vi "ConfigureSimulatedData.vi"() -> ()   [LabVIEW 2017, in "IrAcquisition.lvlib"]
uses:
  <vilib>/addons/InsightCM/Devices/Shared/Ir/IrAcquisition/IrAcquisition.lvlib
  <vilib>/addons/InsightCM/Devices/Shared/Ir/IrAcquisition/controls/simScaleConfig.ctl
  <vilib>/addons/InsightCM/Devices/Shared/Ir/IrAcquisition/subVIs/SimConfigGlobal.vi
panel:
  in  "Camera 2 Data":string(combo)
  in  "Camera 2 SN":string="67890DEF"
  in  "Camera 2 Config":T1={"Max"={"Enable"=FALSE, "New Max Temp"=100.0, "KeepMin"=FALSE}, "Noise"={"Randomize"=TRUE, "Max delta"=0.5}, "Hotspot"={"hotspot"=FALSE, "Rectangle"={"left"=100, "top"=200, "right"=150, "bottom"=250}, "Temperature"=100.0}}
  in  "Camera 1 Data":string(combo)
  in  "Camera 1 SN":string="12345ABC"
  in  "Camera 1 Config":T1={"Max"={"Enable"=FALSE, "New Max Temp"=100.0, "KeepMin"=FALSE}, "Noise"={"Randomize"=TRUE, "Max delta"=0.5}, "Hotspot"={"hotspot"=FALSE, "Rectangle"={"left"=100, "top"=200, "right"=150, "bottom"=250}, "Temperature"=100.0}}
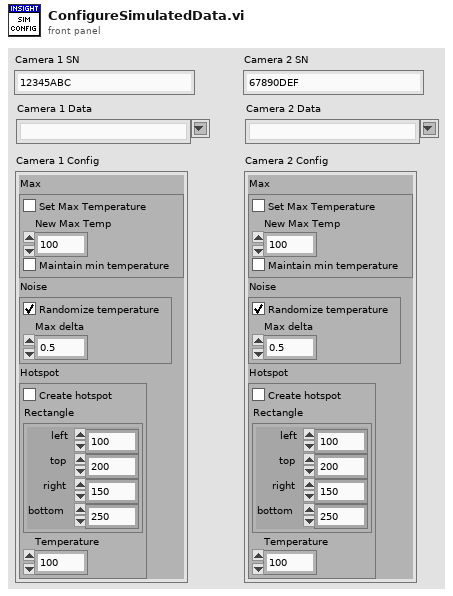
[diagram p1: front panel]
types:
  T1 = typedef "IrAcquisition.lvlib/simScaleConfig.ctl" = cluster{"Max":cluster{"Enable":bool, "New Max Temp":sgl, "KeepMin":bool}, "Noise":cluster{"Randomize":bool, "Max delta":sgl}, "Hotspot":cluster{"hotspot":bool, "Rectangle":cluster{"left":i16, "top":i16, "right":i16, "bottom":i16}, "Temperature":sgl}}
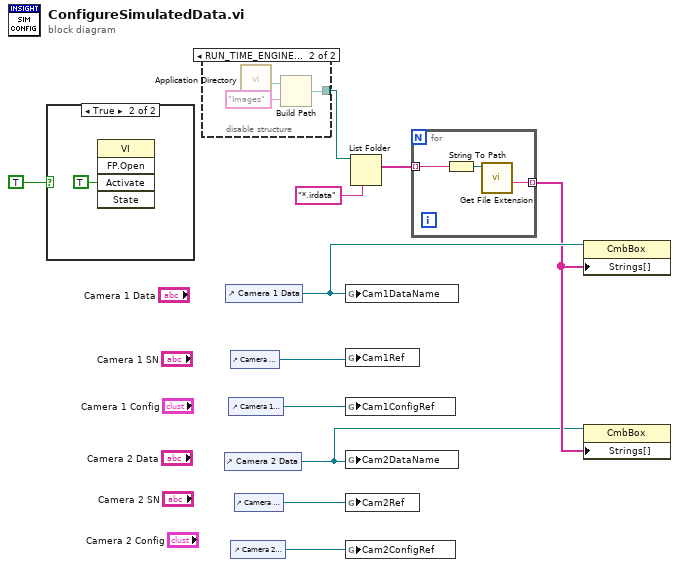
[diagram p0: block diagram]
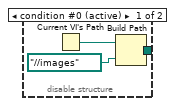
[diagram p2: hidden frame]
diagram:
  n1 = case shown="True" TRUE {
    frame False {
    }
    frame True {
      n2 = invoke class="VI" method="FP.Open"("Activate"=TRUE ("Activate?")) -> ()  [unwired: 4 in, 5 out]
    }
  }
  n3 = disable-structure shown="RUN_TIME_ENGINE==True" {
    disable-tunnel: [w13 w16] -> w8
    frame condition #0 (active) {
      n4 = Current VI's Path() -> (path=w15:path)
      n5 = Build Path(base path=w15, name or relative path=path "../../images" ("path")) -> (appended path=w13:path)
    }
    frame condition #1 {
      n6 = call <vilib>:"Application Directory.vi"() -> ("Application Directory"=w18:path)
      n7 = Build Path(base path=w18, name or relative path="Images") -> (appended path=w16:path)
    }
  }
  n8 = control-ref of="Camera 2 Data"() -> (w3:refnum<vi>)
  n9 = control-ref of="Camera 1 Data"() -> (w5:refnum<vi>)
  n10 = control-ref of="Camera 1 Config"() -> (w9:refnum<vi>)
  n11 = control-ref of="Camera 1 SN"() -> (w10:refnum<vi>)
  n12 = control-ref of="Camera 2 Config"() -> (w1:refnum<vi>)
  n13 = control-ref of="Camera 2 SN"() -> (w2:refnum<vi>)
  n14 = global write "SimConfigGlobal.vi" "Cam1DataName"(w5) -> ()
  n15 = global write "SimConfigGlobal.vi" "Cam1Ref"(w10) -> ()
  n16 = global write "SimConfigGlobal.vi" "Cam1ConfigRef"(w9) -> ()
  n17 = global write "SimConfigGlobal.vi" "Cam2DataName"(w3) -> ()
  n18 = global write "SimConfigGlobal.vi" "Cam2Ref"(w2) -> ()
  n19 = global write "SimConfigGlobal.vi" "Cam2ConfigRef"(w1) -> ()
  n20 = List Folder(path=w8, pattern="*.irdata") -> (filenames=w6:string[])  [unwired: 2 in, 3 out]
  n21 = for {
    tunnel: w6 -> [w21] mode=indexing
    tunnel: [w19] -> w4 mode=indexing
    n22 = String To Path(string=w21) -> (path=w20:path)
    n23 = call <vilib>:"Get File Extension.vi"("file"=w20) -> ("filename without extension"=w19:string)  [unwired: 6 in, 4 out]
  }
  n24 = property class="CmbBox"(reference=w5, "Strings[]"=w4) -> ()  [unwired: 1 in, 2 out]
  n25 = property class="CmbBox"(reference=w3, "Strings[]"=w4) -> ()  [unwired: 1 in, 2 out]
